vi "Project mu.vi"() -> ()   [LabVIEW 2023]
uses:
  <vilib>/DAQmx/read.llb/DAQmx Read (Analog 2D DBL NChan NSamp).vi
  <vilib>/Analysis/baseanly.llb/Mean (DBL).vi
  <vilib>/DAQmx/create/channels.llb/DAQmx Create Channel (AI-Voltage-Basic).vi
  <vilib>/DAQmx/create/channels.llb/DAQmx Create Channel (AI-Voltage-Custom with Excitation).vi
  <vilib>/DAQmx/configure/timing.llb/DAQmx Timing (Sample Clock).vi
  <vilib>/DAQmx/configure/trigger.llb/DAQmx Start Trigger (Analog Edge).vi
  <vilib>/DAQmx/miscellaneous.llb/DAQmx Fill In Error Info.vi
  <vilib>/Analysis/NI_AALPro.lvlib
  <vilib>/Analysis/NI_AALBase.lvlib
panel:
  out "Coefficient of dynamic friction vs. Time Graph":cluster{dbl[], dbl[]}(graph)
  out "Mass (kg)":dbl
  in  "Test File Path":path
  in  "Test Number":dbl=1.0 min=1.0 format="%#_1f"
  out "Tension in string (N)":dbl
  in  "Seconds Per Loop":dbl
  out "Coefficient  of static friction":dbl
  out "Acceleration (m/s^2)":dbl
  out "Velocity (m/s)":dbl
  out "Coefficient of kinematic friction":dbl
  out "Normal force (N)":dbl
  out "Frictional force (N)":dbl
  out "Load vs. Time Graph":cluster{dbl[], dbl[]}(graph)
  out "Load (N) vs. Displacement (mm) Graph":cluster{dbl[], dbl[]}(graph)
  out "Displacement mm vs. Time (s) Graph":cluster{dbl[], dbl[]}(graph)
  in  "Triggering system":bool
  in  "Load  Scale:":tag
  in  "Load DAQ Channel":tag
  in  "Load description":string="Pounds - lbf"
  in  "Initial displacement (mm)":dbl
  in  "Displacement  Description":string="Positon- inches"
  in  "Sample mode":i32(ring)=10178 items=["Finite Samples"=10178, "Continuous Samples"=10123, "Hardware Timed Single Point"=12522]
  in  "DAQ Rate":dbl=5000.0
  in  "stop":bool
  in  "# Loops":i32
  in  "Displacement custom scale":tag="LaserDicplacement (mm)(ST06)(Monday)"
  in  "Dispalcement channel":tag="cDAQ2Mod1/ai0"
  # "WE WOULD LIKE TO APPRECIATE THE PROFESSOR AND GAs FOR THEIR HELP AND SUPPORT THROUGHT THIS COURsE"
  # "GROUP 8"
  # "PROJECT MU 2"
  # "GRAPHS"
  # "DAQ Input"
  # "File information"
  # "CALCULATED VALUES"
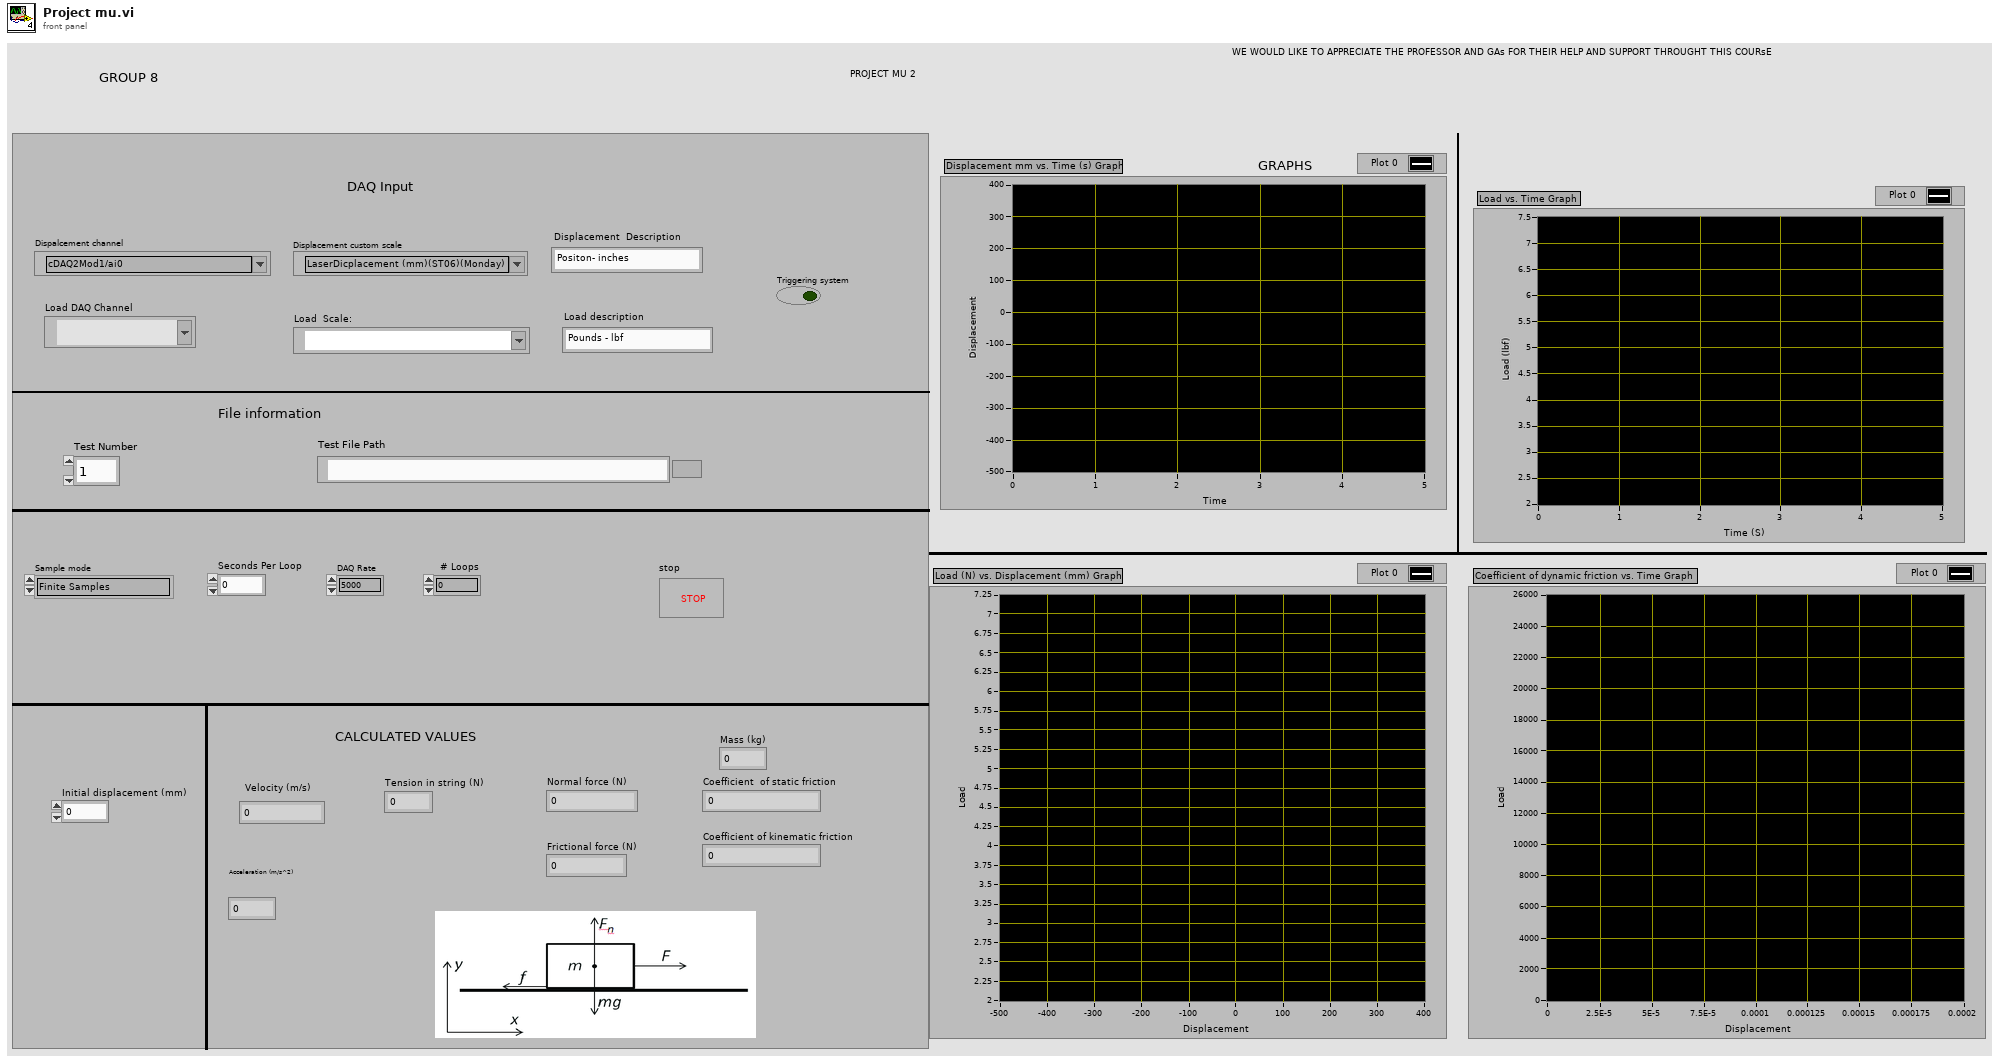
[diagram p1: front panel]
types:
  T1 = enum16{"open", "replace", "create", "open or create", "replace or create", "replace or create with confirmation"}
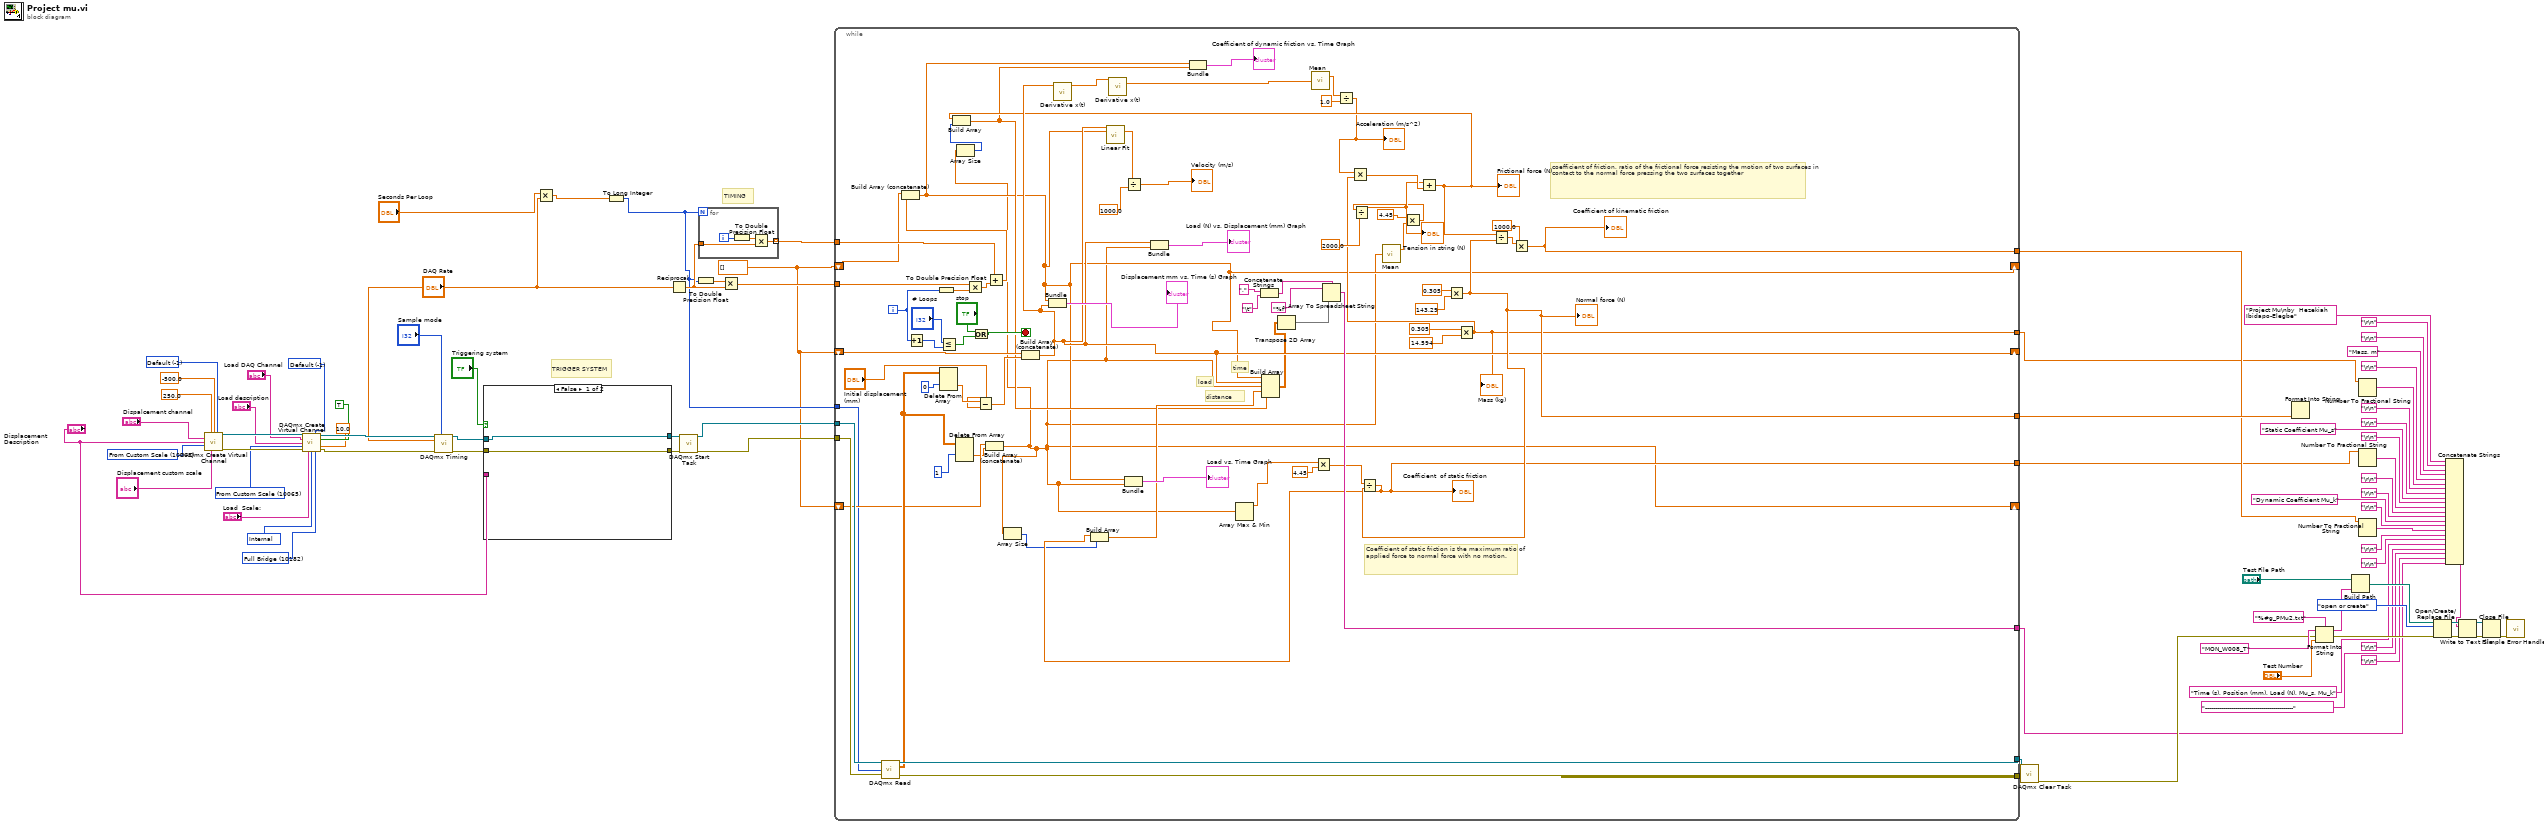
[diagram p0: block diagram]
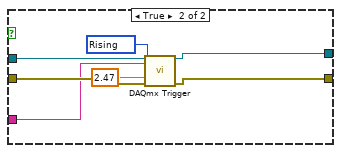
[diagram p2: hidden frame]
diagram:
  w56 = 10065 items=["Volts"=10348, "From Custom Scale"=10065] ("units")
  w57 = 10200 items=["Internal"=10200, "External"=10167, "None"=10230] ("voltage excitation source")
  w58 = 10182 items=["Full Bridge"=10182, "Half Bridge"=10187, "Quarter Bridge"=10270, "No Bridge"=10228] ("bridge configuration")
  w62 = -1 items=["Default"=-1, "RSE"=10083, "NRSE"=10078, "Differential"=10106, "Pseudodifferential"=12529] ("input terminal configuration")
  w1 = dbl[] []
  w77 = 10065 items=["Volts"=10348, "From Custom Scale"=10065] ("units")
  w79 = -1 items=["Default"=-1, "RSE"=10083, "NRSE"=10078, "Differential"=10106, "Pseudodifferential"=12529] ("input terminal configuration")
  # "TRIGGER SYSTEM"
  # "TIMING"
  n1 = call-poly <vilib>:"DAQmx Create Virtual Channel.vi"("maximum value"=250.0, "minimum value"=-500.0, "input terminal configuration"=w79, "physical channels"="Dispalcement channel", "name to assign"="Displacement  Description", "units"=w77, "custom scale name"="Displacement custom scale") -> ("task out"=w68:refnum<k21>, "error out"=w66:errorcluster)  [unwired: 7 in]
  n2 = call-poly <vilib>:"DAQmx Create Virtual Channel.vi"("task in"=w68, "input terminal configuration"=w62, "physical channels"="Load DAQ Channel", "use excitation for scaling"=TRUE, "name to assign"="Load description", "units"=w56, "voltage excitation value"=10.0, "error in"=w66, "custom scale name"="Load  Scale:", "voltage excitation source"=w57, "bridge configuration"=w58) -> ("task out"=w67:refnum<k21>, "error out"=w65:errorcluster)  [unwired: 3 in]
  n3 = call-poly <vilib>:"DAQmx Timing.vi"("task/channels in"=w67, "sample mode"="Sample mode", "rate"="DAQ Rate", "error in"=w65) -> ("task out"=w55:refnum<k21>, "error out"=w52:errorcluster)  [unwired: 10 in]
  n4 = case shown="False" "Triggering system" {
    tunnel: w55 -> [w83 w89]
    tunnel: [w83 w88] -> w54
    tunnel: w52 -> [w82 w87]
    tunnel: [w82 w86] -> w51
    tunnel: "Displacement  Description" -> [_ w84]
    frame False {
    }
    frame True {
      w90 = 10280 items=["Rising"=10280, "Falling"=10171] ("slope")
      n5 = call-poly <vilib>:"DAQmx Trigger.vi"("task/channels in"=w89, "source"=w84, "slope"=w90, "level"=2.47, "error in"=w87) -> ("task out"=w88:refnum<k21>, "error out"=w86:errorcluster)  [unwired: 9 in]
    }
  }
  n6 = Multiply(x="Seconds Per Loop", y="DAQ Rate") -> (x*y=w44:dbl)
  n7 = To Long Integer(number=w44) -> (32bit integer=w43:i32)
  n8 = Reciprocal(x="DAQ Rate") -> (1/x=w73:dbl)
  n9 = call <vilib>:"DAQmx Start Task.vi"("task/channels in"=w54, "error in"=w51) -> ("task out"=w53:refnum<k21>, "error out"=w50:errorcluster)  [unwired: 12 in]
  n10 = To Double Precision Float(number=w43) -> (double precision float=w75:dbl)
  n11 = for {
    N: w43 -> [_]
    tunnel: w73 -> [w92]
    tunnel: [w91] -> w72 mode=indexing
    i -> [w94]
    n12 = To Double Precision Float(number=w94) -> (double precision float=w93:dbl)
    n13 = Multiply(x=w93, y=w92) -> (x*y=w91:dbl)
  }
  n14 = Multiply(x=w75, y=w73) -> (x*y=w74:dbl)
  n15 = while {
    shift-right: [w123] -> _
    shift-left: w1 -> [w157]
    shift-right: [w109] -> _
    shift-left: w1 -> [w150]
    tunnel: w74 -> [w158]
    tunnel: w72 -> [w156]
    tunnel: [w154] -> w70
    tunnel: [w153] -> w69
    tunnel: w50 -> [w148]
    tunnel: w53 -> [w147]
    shift-right: [w101] -> _
    shift-left: w1 -> [w140]
    tunnel: [w128] -> w47
    tunnel: w43 -> [w127]
    tunnel: [w124] -> w5
    tunnel: [w95] -> w4
    tunnel: [w118] -> w3
    tunnel: [w111] -> w2
    i -> [w159]
    stop <- w163 stop-if-true
    # "coefficient of friction, ratio of the frictional force resisting the motion of two surfaces in contact to the normal force pressing the two surfaces together"
    # "Coefficient of static friction is the maximum ratio of applied force to normal force with no motion."
    # "load"
    # "time"
    # "distance"
    n16 = call-poly <vilib>:"DAQmx Read.vi"("task/channels in"=w147, "number of samples per channel"=w127, "error in"=w148) -> ("task out"=w154:refnum<k21>, "data"=w145:dbl[][], "error out"=w153:errorcluster)  [unwired: 10 in]
    n17 = Increment(x=w159) -> (x+1=w161:i32)
    n18 = To Double Precision Float(number=w159) -> (double precision float=w166:dbl)
    n19 = Delete From Array(array=w145, index (row)=0) -> (deleted portion=w143:dbl[])  [unwired: 2 in, 1 out]
    n20 = Less Or Equal?(x="# Loops", y=w161) -> (x <= y?=w160:bool)
    n21 = Delete From Array(array=w145, index (row)=1) -> (deleted portion=w132:dbl[])  [unwired: 2 in, 1 out]
    n22 = Multiply(x=w158, y=w166) -> (x*y=w165:dbl)
    n23 = Or(x="stop", y=w160) -> (x .or. y?=w163:bool)
    n24 = Subtract(x=w143, y="Initial displacement (mm)") -> (x-y=w141:dbl[])
    n25 = Build Array (concatenate)(w140, w132) -> (w101:dbl[])
    n26 = Array Size(array=w101) -> (size(s)=w115:i32)
    n27 = Add(x=w156, y=w165) -> (x+y=w149:dbl[])
    n28 = Build Array (concatenate)(w150, w149) -> (w109:dbl[])
    n29 = Array Size(array=w101) -> (size(s)=w117:i32)
    n30 = Build Array (concatenate)(w157, w141) -> (w123:dbl[])
    n31 = Bundle(w109, w123) -> (→"Displacement mm vs. Time (s) Graph":cluster{dbl[], dbl[]})  [unwired: 1 in]
    n32 = call <vilib>:"Derivative x(t).vi"("X"=w123) -> ("dX/dt"=w126:dbl[])  [unwired: 9 in, 1 out]
    n33 = call <vilib>:"Linear Fit.vi"("Y"=w123, "X"=w109) -> ("slope"=w130:dbl)  [unwired: 9 in, 4 out]
    n34 = call <vilib>:"Derivative x(t).vi"("X"=w126) -> ("dX/dt"=w134:dbl[])  [unwired: 9 in, 1 out]
    n35 = Bundle(w109, w101) -> (→"Load vs. Time Graph":cluster{dbl[], dbl[]})  [unwired: 1 in]
    n36 = Divide(x=w130, y=1000.0) -> (x/y=→"Velocity (m/s)":dbl)
    n37 = Bundle(w123, w101) -> (→"Load (N) vs. Displacement (mm) Graph":cluster{dbl[], dbl[]})  [unwired: 1 in]
    n38 = Array Max & Min(array=w101) -> (max value=w99:dbl)  [unwired: 3 out]
    n39 = Concatenate Strings("," ("delimiter (Tab)"), "\t") -> (w106:string)
    n40 = call-poly <vilib>:"Mean.vi"("X"=w134) -> ("mean"=w114:dbl)  [unwired: 1 out]
    n41 = Multiply(x=w99, y=4.45) -> (x*y=w98:dbl)
    n42 = Divide(x=w114, y=1.0) -> (x/y=w112:dbl)
    "Acceleration (m/s^2)" <- w112
    n43 = call-poly <vilib>:"Mean.vi"("X"=w101) -> ("mean"=w102:dbl)  [unwired: 1 out]
    n44 = Multiply(x=4.45, y=w102) -> (x*y=w103:dbl)
    n45 = Divide(x=w103, y=2000.0) -> (x/y=w125:dbl)
    "Tension in string (N)" <- w125
    n46 = Multiply(x=0.305, y=143.29) -> (x*y=w128:dbl)
    "Normal force (N)" <- w128
    n47 = Divide(x=w98, y=w128) -> (x/y=w118:dbl)
    "Coefficient  of static friction" <- w118
    n48 = Build Array(w118, w117) -> (w120:dbl[])
    n49 = Multiply(x=0.305, y=14.594) -> (x*y=w111:dbl)
    "Mass (kg)" <- w111
    n50 = Multiply(x=w112, y=w111) -> (x*y=w133:dbl)
    n51 = Add(x=w125, y=w133) -> (x+y=w116:dbl)
    "Frictional force (N)" <- w116
    n52 = Build Array(w116, w115) -> (w110:dbl[])
    n53 = Bundle(w109, w110) -> (→"Coefficient of dynamic friction vs. Time Graph":cluster{dbl[], dbl[]})  [unwired: 1 in]
    n54 = Build Array(w109, w123, w101, w120, w110) -> (w119:dbl[][])
    n55 = Transpose 2D Array(2D array=w119) -> (transposed array=w151:dbl[][])
    n56 = Array To Spreadsheet String(delimiter (Tab)=w106, array=w151, 3:"%f" ("format string")) -> (spreadsheet string=w124:string)
    n57 = Divide(x=w116, y=w128) -> (x/y=w96:dbl)
    n58 = Multiply(x=w96, y=1000.0) -> (x*y=w95:dbl)
    "Coefficient of kinematic friction" <- w95
  }
  n59 = call <vilib>:"DAQmx Clear Task.vi"("task in"=w70, "error in"=w69) -> ("error out"=w6:errorcluster)  [unwired: 13 in]
  n60 = Format Into String(w47) -> ()  [unwired: 3 in, 2 out]
  n61 = Format Into String(format string="%#g_PMu2.txt", initial string="MON_W008_T" ("format string"), error in=w6, "Test Number") -> (resulting string=w31:string, error out=w29:errorcluster)
  n62 = Build Path(base path="Test File Path", name or relative path=w31) -> (appended path=w35:path)
  n63 = Number To Fractional String(number=w2) -> (F-format string=w23:string)  [unwired: 3 in]
  n64 = Number To Fractional String(number=w3) -> (F-format string=w18:string)  [unwired: 3 in]
  n65 = Number To Fractional String(number=w4) -> (F-format string=w13:string)  [unwired: 3 in]
  n66 = Open/Create/Replace File(file path (use dialog)=w35, error in=w29, operation (0:open)=T1."open or create") -> (refnum out=w41:refnum<file>, error out=w38:errorcluster)  [unwired: 3 in, 1 out]
  n67 = Concatenate Strings("Project Mu\nby  Hezekiah Ibidapo-Elegbe" ("string"), "\r\n", "\r\n", "Mass, m" ("string"), "\r\n" ("string"), w23, "\r\n" ("string"), "\r\n" ("string"), "Static Coefficient Mu_s" ("string"), "\r\n" ("string"), w18, "\r\n" ("string"), "\r\n" ("string"), "Dynamic Coefficient Mu_k" ("string"), "\r\n" ("string"), w13, "\r\n" ("string"), "\r\n" ("string"), "Time (s), Position (mm), Load (N), Mu_s, Mu_k" ("string"), "\r\n" ("string"), "--------------------------------------------" ("string"), "\r\n" ("string"), w5) -> (w40:string)
  n68 = Write to Text File(file (use dialog)=w41, text=w40, error in=w38) -> (refnum out=w39:refnum<file>, error out=w37:errorcluster)  [unwired: 1 in, 1 out]
  n69 = Close File(refnum=w39, error in=w37) -> (error out=w34:errorcluster)  [unwired: 1 out]
  n70 = call <vilib>:"Simple Error Handler.vi"("error in (no error)"=w34) -> ()  [unwired: 4 in, 5 out]
